vi "Select File Group Channel.vi"(8 "error in (no error)":errorcluster, 9 "File-group-channel Y":T1(array[cluster]), 10 "File-group-channel X":T1(array[cluster]), 11 "MagLabGraph in":refnum<class "XY Plot.lvclass">) -> (0 "error out":errorcluster, 3 "MagLabGraph out":refnum<class "XY Plot.lvclass">)   [LabVIEW 2015, in "XY Plot.lvclass"]
uses:
  XY Plot.lvclass
  XY Plot.lvclass/XY Plot.ctl
  NHMFL_Core/Libraries/Utilities/Controls/Plot Indexes.ctl
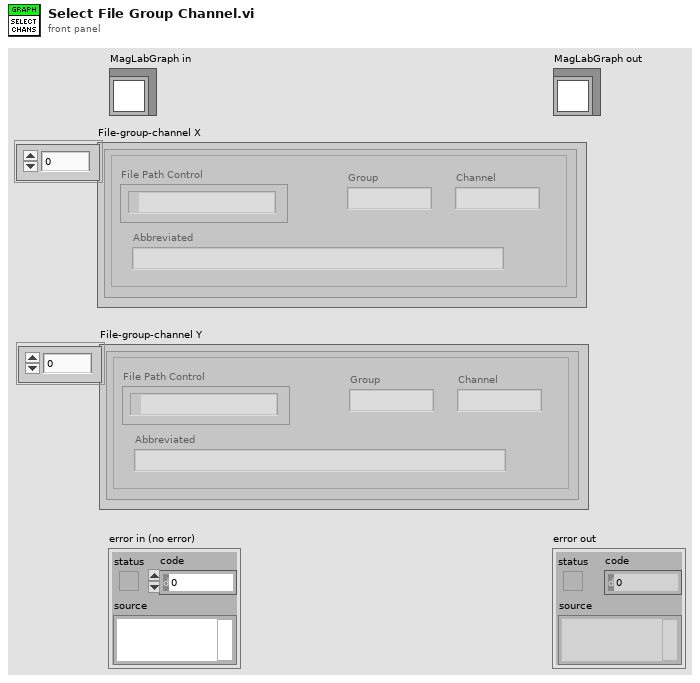
[diagram p1: front panel]
types:
  T1 = cluster{"File Path Control":path, "Group":string, "Channel":string, "Abbreviated":string}[]
  T2 = typedef "Plot Indexes.ctl" = cluster{"X":u16, "Y":u16}
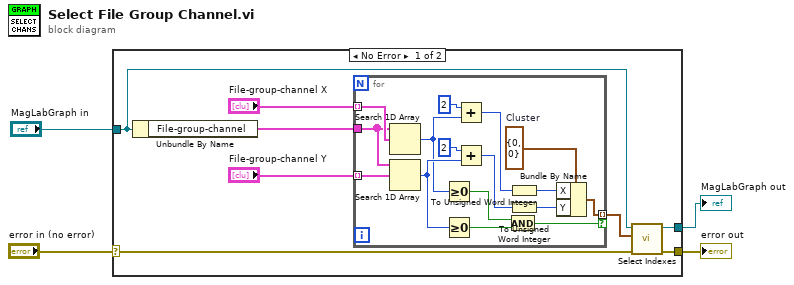
[diagram p0: block diagram]
diagram:
  n1 = case shown="No Error" "error in (no error)" {
    selector: "error in (no error)" -> [w7 w30]
    tunnel: [w6 w30] -> w3
    tunnel: [w8 w29] -> w1
    tunnel: "MagLabGraph in" -> [w9 w29]
    frame No Error {
      n2 = Unbundle By Name(w9) -> ("File-group-channel"=w10:T1)
      n3 = for {
        tunnel: "File-group-channel X" -> [w28] mode=indexing
        tunnel: "File-group-channel Y" -> [w27] mode=indexing
        tunnel: w10 -> [w26]
        tunnel: [w22] -> w5 mode=indexing if=w21
        w25 = T2 {"X"=0, "Y"=0}  # Cluster
        n4 = Search 1D Array(1D array=w26, element=w28) -> (index of element=w15:i32)  [unwired: 1 in]
        n5 = Search 1D Array(1D array=w26, element=w27) -> (index of element=w18:i32)  [unwired: 1 in]
        n6 = Greater Or Equal To 0?(x=w15) -> (x >= 0?=w24:bool)
        n7 = Greater Or Equal To 0?(x=w18) -> (x >= 0?=w23:bool)
        n8 = Add(x=2, y=w15) -> (x+y=w14:i32)
        n9 = Add(x=2, y=w18) -> (x+y=w17:i32)
        n10 = And(x=w24, y=w23) -> (x .and. y?=w21:bool)
        n11 = To Unsigned Word Integer(number=w14) -> (unsigned 16bit integer=w13:u16)
        n12 = To Unsigned Word Integer(number=w17) -> (unsigned 16bit integer=w16:u16)
        n13 = Bundle By Name(cluster=w25, "X"=w13, "Y"=w16) -> (w22:T2)
      }
      n14 = call-dynamic "Select Indexes.vi"("error in (no error)"=w7, "Plot Indexes Array"=w5, "MagLabGraph in"=w9) -> ("error out"=w6:errorcluster, "MagLabGraph out"=w8:refnum<class "XY Plot.lvclass">)  [unwired: 7 in]
    }
    frame Error {
    }
  }
  "error out" <- w3
  "MagLabGraph out" <- w1
